vi "2. 初始化：光纤起点.vi"(11 "初始偏移量：相对于起点(14,27)":dbl[](array[numeric])=[0.0, 0.0]) -> (3 "坐标原点 重新选定后 的 一维数组":dbl[](array[numeric]))   [LabVIEW 2018]
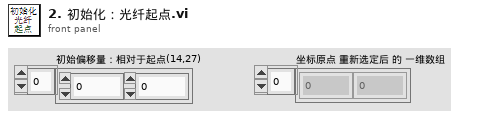
[diagram p1: front panel]
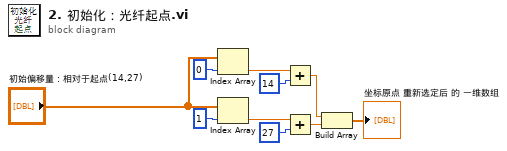
[diagram p0: block diagram]
diagram:
  n1 = Index Array(array="初始偏移量：相对于起点(14,27)", index=0) -> (element=w5:dbl)
  n2 = Index Array(array="初始偏移量：相对于起点(14,27)", index=1) -> (element=w4:dbl)
  n3 = Add(x=w5, y=14) -> (x+y=w8:dbl)
  n4 = Add(x=w4, y=27) -> (x+y=w9:dbl)
  n5 = Build Array(w8, w9) -> (→"坐标原点 重新选定后 的 一维数组":dbl[])
